vi "Stop Core.vi"(10 "final error code":i32, 11 "IED in":refnum<class "IED.lvclass">) -> (3 "IED out":refnum<class "IED.lvclass">)   [LabVIEW 2018, in "IED Actor.lvlib" / "IED.lvclass"]
doc: "(<B>Filename</B>: Actor Framework.lvlib:Actor.lvclass:Stop Core.vi)\n\nDefines what the actor does before it stops. Use the <B>final error code</B> input to determine whether the actor shut down in response to an error.\n\nBy default, this method does nothing. A descendant class may override it to define behavior, such as shutting down any processes the actor initiated in its override of the Actor Core method."
uses:
  IED.lvclass
  C:/Users/Administrator/Desktop/2018LabVIEW EMS/IED Actors/Device DDS Communications Framework/Device DDS Communications/Device DDS Communications.lvclass
  Device DDS Communications Framework/Device DDS Communications/Device DDS Communications.lvclass/Device DDS Communications.ctl
  <vilib>/ORNL/CSEISMIC DDS/CSEISMIC DDS Base/Data Types/IED_setMicrogridID.ctl
  <vilib>/ORNL/CSEISMIC DDS/CSEISMIC DDS Base/Data Types/Controls/DeviceID.ctl
  <vilib>/ORNL/CSEISMIC DDS/CSEISMIC DDS Base/CSEISMIC DDS.lvclass/CSEISMIC DDS.ctl
  <vilib>/ORNL/CSEISMIC DDS/CSEISMIC DDS Base/Accessors/Read DDS Reference.vi
  <vilib>/ORNL/CSEISMIC DDS/DDS Writer/DDS Writer.lvclass
  C:/Program Files (x86)/National Instruments/LabVIEW 2018/vi.lib/ORNL/CSEISMIC DDS/CSEISMIC DDS Base/CSEISMIC DDS.lvclass
  <vilib>/ORNL/CSEISMIC DDS/CSEISMIC DDS Base/Error Handler.vi
  Device DDS Communications Framework/Device DDS Communications/Device DDS Communications.lvclass
  <vilib>/ORNL/CSEISMIC DDS/CSEISMIC DDS Base/CSEISMIC DDS.lvclass
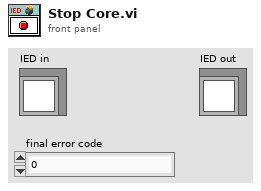
[diagram p1: front panel]
types:
  T1 = typedef "CSEISMIC DDS.lvlib/CSEISMIC DDS.lvclass/DeviceID.ctl" = string
  T2 = typedef "CSEISMIC DDS.lvlib/CSEISMIC DDS.lvclass/IED_setMicrogridID.ctl" = cluster{"DeviceID":T1, "MicrogridID":u8}
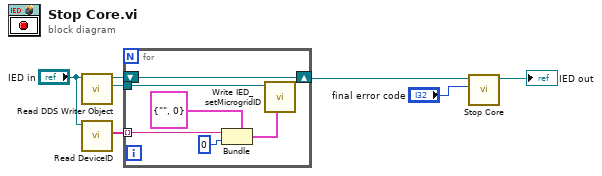
[diagram p0: block diagram]
diagram:
  n1 = call "Read DDS Writer Object.vi"("Device DDS Communications in"="IED in") -> ("DDS Writer Object"=w3:refnum<class "DDS Writer.lvclass">, "Device DDS Communications out"=w2:refnum<class "IED.lvclass">)  [unwired: 9 in]
  n2 = call-dynamic "Read DeviceID.vi"("Device DDS Communications in"="IED in") -> ("DeviceID"=w5:T1[])  [unwired: 9 in, 1 out]
  n3 = for {
    tunnel: w5 -> [w12] mode=indexing
    tunnel: w3 -> [w11]
    shift-right: [w8] -> w1
    shift-left: w2 -> [w8]
    n4 = Bundle(cluster=T2 {"DeviceID"="", "MicrogridID"=0} ("Cluster"), "DeviceID"=w12, "MicrogridID"=u8 0) -> (w10:T2)
    n5 = call <vilib>:"Write IED_setMicrogridID.vi"("IED_setMicrogridID"=w10, "DDS Writer in"=w11) -> ()  [unwired: 8 in, 2 out]
  }
  n6 = call-parent "Stop Core.vi"("final error code"="final error code", "Device DDS Communications in"=w1) -> ("Device DDS Communications out"=→"IED out":refnum<class "IED.lvclass">)  [unwired: 9 in]
